vi "daqio_Create_Tag_Type.vi"(6 "new Tag default value":string, 7 "new Tag  Data Type":string(combo)="string", 8 "error in (no error)":errorcluster, 9 "new Tag Label":string, 10 "new Tag Key":string, 11 "daq.io type in":T1={"daq.io ref"=refnum, "daq.io API Base"="http://dashboard.daq.io/api/v1", "Device Type Key"="", "Device Key"="", "Account ID"=""}) -> (0 "error out":errorcluster, 1 "JSON string":string, 2 "actual Tag Key written":string, 3 "daq.io type out":T1={"daq.io ref"=refnum, "daq.io API Base"="http://dashboard.daq.io/api/v1", "Device Type Key"="", "Device Key"="", "Account ID"=""})   [LabVIEW 2013, in "daqio minimal.lvlib"]
doc: "This VI creates a new Tag definition (Tag Type), so Tags of this type can be used in the future. When automatic error checking is required, consider using \"Check and autocreate Tag\""
uses:
  daqio minimal.lvlib
  _typedefs/daqio-Type.ctl
  <vilib>/httpClient/ClientHandle.ctl
  <vilib>/Easy HTTP Client/Easy HTTP.lvlib
  <vilib>/httpClient/LabVIEWHTTPClient.lvlib
panel:
  out "body":string
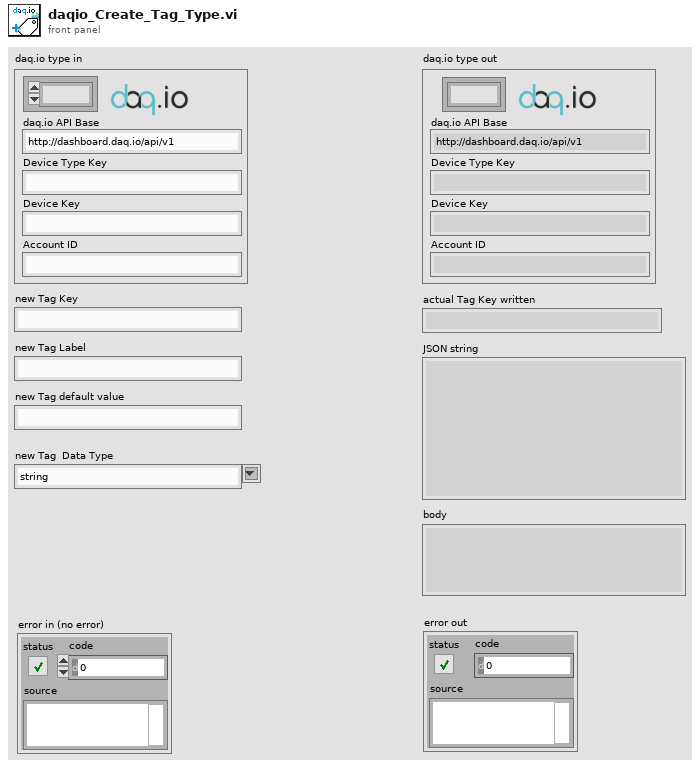
[diagram p1: front panel]
types:
  T1 = typedef "daqio minimal.lvlib/daqio-Type.ctl" = cluster{"daq.io ref":T2, "daq.io API Base":string, "Device Type Key":string, "Device Key":string, "Account ID":string}
  T2 = typedef "LabVIEWHTTPClient.lvlib/ClientHandle.ctl" = refnum<k1>
  T3 = cluster{"label":string, "device_type_id":string, "default":string, "key":string, "data_type":string}
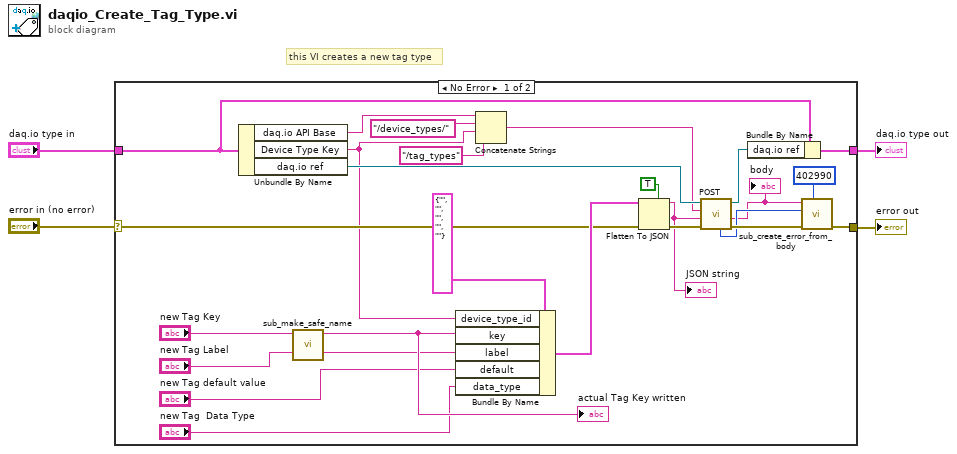
[diagram p0: block diagram]
diagram:
  # "this VI creates a new tag type"
  n1 = case shown="No Error" "error in (no error)" {
    selector: "error in (no error)" -> [w25 w30]
    tunnel: [w22 w31] -> w4
    tunnel: [w8 w30] -> w3
    tunnel: "daq.io type in" -> [w21 w31]
    frame No Error {
      n2 = Unbundle By Name(w21) -> ("daq.io API Base"=w13:string, "Device Type Key"=w17:string, "daq.io ref"=w24:T2)
      n3 = call "sub_make_safe_name.vi"("Input String"="new Tag Key") -> ("Safe Output String"=w16:string)  [unwired: 10 in]
      "actual Tag Key written" <- w16
      n4 = Bundle By Name(cluster=T3 {"label"="", "device_type_id"="", "default"="", "key"="", "data_type"=""} ("value"), "device_type_id"=w17, "key"=w16, "label"="new Tag Label", "default"="new Tag default value", "data_type"="new Tag  Data Type") -> (w29:T3)
      n5 = Concatenate Strings(w13, "/device_types/" ("string"), w17, "/tag_types" ("string")) -> (w19:string)
      n6 = Flatten To JSON(enable LabVIEW extensions? (T)=TRUE, anything=w29, error in (no error)=w25) -> (JSON string=w18:string, 11:w23:errorcluster)
      "JSON string" <- w18
      n7 = call <vilib>:"POST.vi"("error in (no error)"=w23, "data"=w18, "url"=w19, "client handle"=w24) -> ("error out"=w9:errorcluster, "body"=w6:string, "client handle out"=w20:T2, "HTTP Response Code"=w7:i32)  [unwired: 3 in, 1 out]
      "body" <- w6
      n8 = Bundle By Name(cluster=w21, "daq.io ref"=w20) -> (w22:T1)
      n9 = call "sub_create_error_from_body.vi"("error code"=402990, "error in (no error)"=w9, "http code"=w7, "body"=w6) -> ("error out"=w8:errorcluster)  [unwired: 7 in]
    }
    frame Error {
    }
  }
  "error out" <- w3
  "daq.io type out" <- w4
